vi "ServiceHostWait.vi"(0 "error in":errorcluster, 2 "Topic":string="/junk", 3 "node":string) -> (1 "Service ROS info out":T1={"topic port"=0, "Node"="", "topic"="", "type"="", "node port"=0, "error "={"status"=FALSE, "code"=0, "source"=""}, "Direction"=enum."Node", "Update (ms)"=1, "FIFO size"=1}, 4 "Request":string)   [LabVIEW 2015]
uses:
  ROS/Code/SubVIs/_ROSControl.ctl
  ROS/Code/SubVIs/_ROSDirection.ctl
  ROS/Code/Console/Servers/ServerSubs/TopicDef.ctl
  ROS/MessageParsing/std_msgs/subs/parse_string_scalar.vi
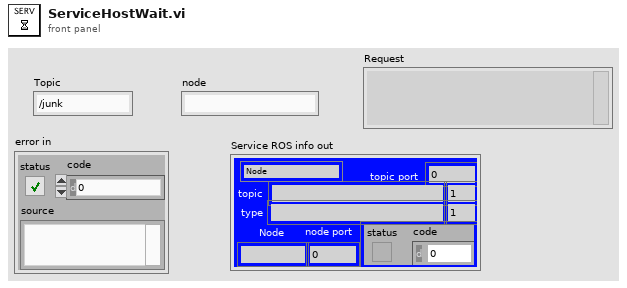
[diagram p1: front panel]
types:
  T1 = typedef "_ROSControl.ctl" = cluster{"topic port":u16, "Node":string, "topic":string, "type":string, "node port":u16, "error ":errorcluster, "Direction":T2, "Update (ms)":u16, "FIFO size":u16}
  T2 = typedef "_ROSDirection.ctl" = enum16{"Node", "Publisher", "Subscriber", "ServiceClient", "ServiceProvider"}
  T3 = typedef "TopicDef.ctl" = cluster{"Topic":string, "Type":string, "Action":T2, "Update (ms)":u16, "queue size":u16}
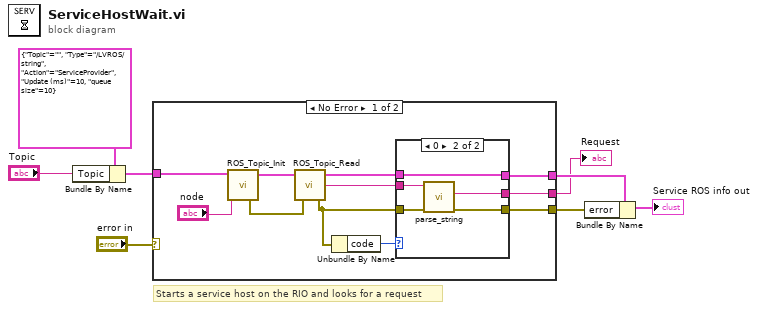
[diagram p0: block diagram]
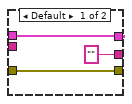
[diagram p2: hidden frame]
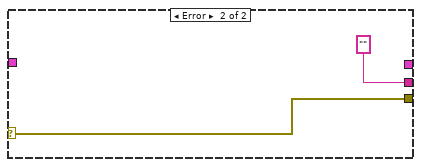
[diagram p3: hidden frame]
diagram:
  # "Starts a service host on the RIO and looks for a request"
  n1 = Bundle By Name(cluster=T3 {"Topic"="", "Type"="/LVROS/string", "Action"=enum."ServiceProvider", "Update (ms)"=10, "queue size"=10} ("Definitions"), "Topic"="Topic") -> (w6:T3)
  n2 = case shown="No Error" "error in" {
    selector: "error in" -> [_ w29]
    tunnel: w6 -> [w18 _]
    tunnel: [w15 w29] -> w4
    tunnel: [w11 _] -> w3
    tunnel: [w9 "" ("msg out")] -> w1
    frame No Error {
      n3 = call "ROS_Topic_Init.vi"("Definitions"=w18, "node"="node") -> ("ROS out"=w17:T1, "error out"=w16:errorcluster)  [unwired: 1 in]
      n4 = call "ROS_Topic_Read.vi"("error in (no error)"=w16, "ROS in"=w17) -> ("error out"=w14:errorcluster, "Reply"=w13:string, "ROS out"=w12:T1)  [unwired: 1 in]
      n5 = Unbundle By Name(w14) -> ("code"=w10:i32)
      n6 = case shown="0" w10 {
        tunnel: [w21 w27] -> w15
        tunnel: w14 -> [w21 w26]
        tunnel: w13 -> [_ w25]
        tunnel: w12 -> [w22 w24]
        tunnel: [w22 w24] -> w11
        tunnel: ["" ("string") w23] -> w9
        frame Default {
        }
        frame 0 {
          n7 = call-poly "parse_string.vi"("error in"=w26, "msg in"=w25) -> ("error out"=w27:errorcluster, "string"=w23:string)  [unwired: 3 in, 1 out]
        }
      }
    }
    frame Error {
    }
  }
  "Request" <- w1
  n8 = Bundle By Name(cluster=w3, "error"=w4) -> (→"Service ROS info out":T1)
